vi "GetConfigurationBasePath.vi"(8 "ErrorIn":errorcluster) -> (0 "ErrorOut":errorcluster, 1 "BasePath":path)   [LabVIEW 2021, in "Application.lvclass"]
uses:
  Application.lvclass
  Interface_TAF_IApplicationConfiguration/IApplicationConfiguration/IApplicationConfiguration.lvclass
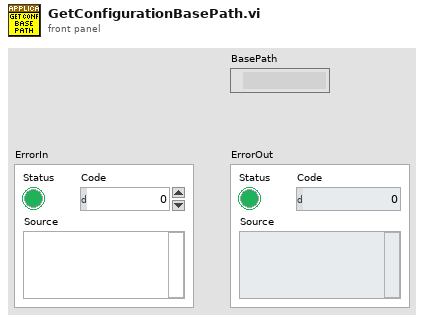
[diagram p1: front panel]
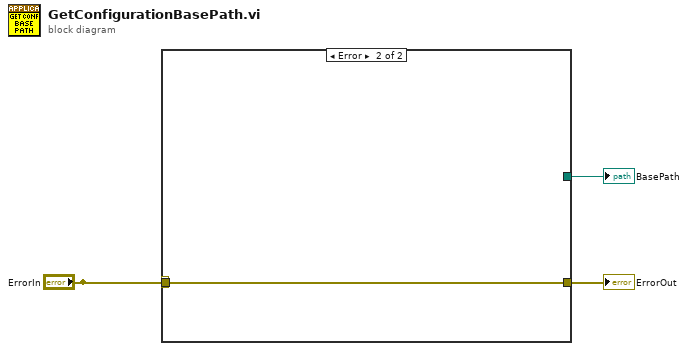
[diagram p0: block diagram]
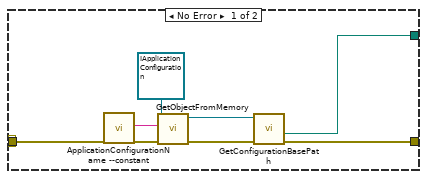
[diagram p2: hidden frame]
diagram:
  n1 = case shown="Error" "ErrorIn" {
    selector: "ErrorIn" -> [w10 w11]
    tunnel: [w8 w11] -> w3
    tunnel: "ErrorIn" -> [_ _]
    tunnel: [w4 _] -> w1
    frame No Error {
      n2 = call "ApplicationConfigurationName --constant.vi"() -> ("AppConfigName"=w6:string)  [unwired: 10 in, 1 out]
      n3 = call "GetObjectFromMemory.vi"("ErrorIn"=w10, "ObjectName"=w6, "Type"=refnum<class "IApplicationConfiguration.lvclass"> refnum ("IApplicationStructure")) -> ("ErrorOut"=w9:errorcluster, "ObjectOut"=w5:refnum<class "IApplicationConfiguration.lvclass">)  [unwired: 7 in]
      n4 = call-dynamic "GetConfigurationBasePath.vi"("ErrorIn"=w9, "ReferenceIn"=w5) -> ("ErrorOut"=w8:errorcluster, "ApplicationBasePath"=w4:path)  [unwired: 7 in, 1 out]
    }
    frame Error {
    }
  }
  "ErrorOut" <- w3
  "BasePath" <- w1
